vi "Set Wrist PID Constants.vi"(8 "error in (no error)":errorcluster, 10 "localConstantSpreadSheet":string[][](array[string]), 11 "robotID":string) -> (0 "error out":errorcluster)   [LabVIEW 2020]
uses:
  2023 Robot Global Data.vi
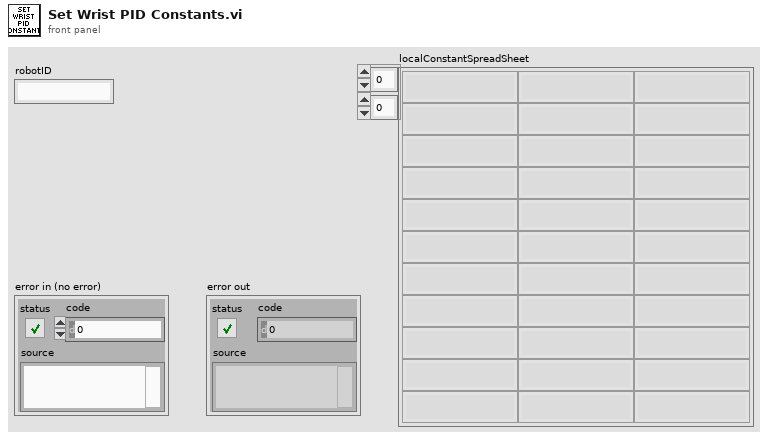
[diagram p1: front panel]
types:
  T1 = cluster{"P Gain":dbl, "I Gain":dbl, "D Gain":dbl, "F Gain":dbl, "I Zone":dbl, "Min Output":dbl, "Max Output":dbl}
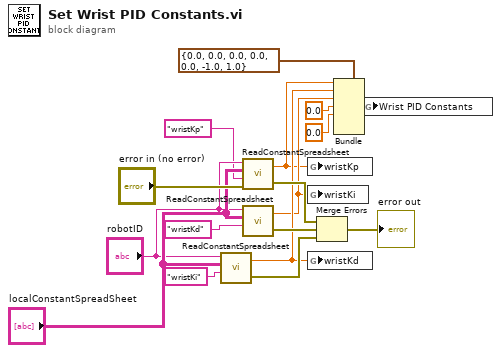
[diagram p0: block diagram]
diagram:
  n1 = call "ReadConstantSpreadsheet.vi"("Constant"="wristKi", "2023ConstantSpreadSheet"="localConstantSpreadSheet", "Robot ID"="robotID") -> ("error out"=w15:errorcluster, "Constant Value"=w12:dbl)  [unwired: 1 in]
  n2 = call "ReadConstantSpreadsheet.vi"("error in"="error in (no error)", "Constant"="wristKp", "2023ConstantSpreadSheet"="localConstantSpreadSheet", "Robot ID"="robotID") -> ("error out"=w13:errorcluster, "Constant Value"=w1:dbl)
  n3 = call "ReadConstantSpreadsheet.vi"("Constant"="wristKd", "2023ConstantSpreadSheet"="localConstantSpreadSheet", "Robot ID"="robotID") -> ("error out"=w14:errorcluster, "Constant Value"=w11:dbl)  [unwired: 1 in]
  n4 = global write "2023 Robot Global Data.vi" "wristKp"(w1) -> ()
  n5 = global write "2023 Robot Global Data.vi" "wristKi"(w11) -> ()
  n6 = global write "2023 Robot Global Data.vi" "wristKd"(w12) -> ()
  n7 = Merge Errors(w13, w14, w15) -> (→"error out":errorcluster)
  n8 = Bundle(cluster=T1 {"P Gain"=0.0, "I Gain"=0.0, "D Gain"=0.0, "F Gain"=0.0, "I Zone"=0.0, "Min Output"=-1.0, "Max Output"=1.0} ("PID Constants"), "P Gain"=w1, "I Gain"=w12, "D Gain"=w11, "F Gain"=0.0, "I Zone"=0.0) -> (w8:T1)  [unwired: 2 in]
  n9 = global write "2023 Robot Global Data.vi" "Wrist PID Constants"(w8) -> ()
